vi "NotARefNum.vi"(3 "reference in":refnum<class "G#Object.lvclass">) -> (0 "not a refnum?":bool, 1 "reference out":refnum<class "G#Object.lvclass">)   [LabVIEW 2017, in "G#Object.lvclass"]
doc: "Checks if the specified object reference is valid."
uses:
  G#Object.lvclass
  G#Object.lvclass/G#Object.ctl
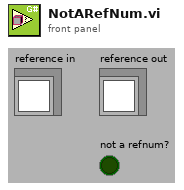
[diagram p1: front panel]
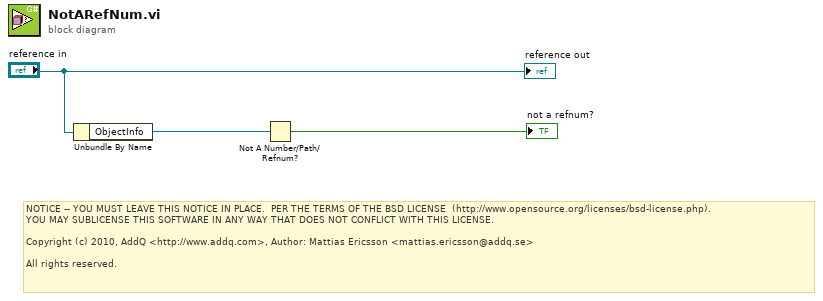
[diagram p0: block diagram]
diagram:
  # "NOTICE -- YOU MUST LEAVE THIS NOTICE IN PLACE.  PER THE TERMS OF THE BSD LICENSE  (http://www.opensource.org/licenses/bsd-license.php).\nYOU MAY SUBLICENSE THIS SOFTWARE IN ANY WAY THAT DOES NOT CONFLICT WITH THIS LICENSE.\n\nCopyright (c) 2010, AddQ <http://www.addq.com>, Author: Mattias Ericsson <mattias.ericsson@addq.se>\n\nAll rights reserved."
  n1 = Unbundle By Name("reference in") -> ("ObjectInfo"=w3:refnum<queue>)
  n2 = Not A Number/Path/Refnum?(number/path/refnum=w3) -> (NaN/Path/Refnum?=→"not a refnum?":bool)
  "reference out" <- "reference in"
